vi "LHF.DB.Mongo.Collection.DropIndex.vi"(8 "error in (no error)":errorcluster, 9 "value":variant, 10 "Collection":string, 11 "LHF.DB.Mongo in":refnum<class "LHF.DB.Mongo.lvclass">) -> (0 "error out":errorcluster, 1 "Ok":bool, 3 "LHF.DB.Mongo out":refnum<class "LHF.DB.Mongo.lvclass">)   [LabVIEW 2013, in "LHF.DB.Mongo.lvclass"]
doc: "Creates an index in collection. Variable name, type & content will be used."
uses:
  LHF.DB.Mongo.lvclass
  C:/Users/Ricardo/Desktop/Projetos/LabVIEW-MongoDB/src/Driver/MongoDB.Driver.dll
  LabVIEW-MongoDB/src/Driver/MongoDB.Driver.dll
  <vilib>/Utility/VariantDataType/VariantType.lvlib
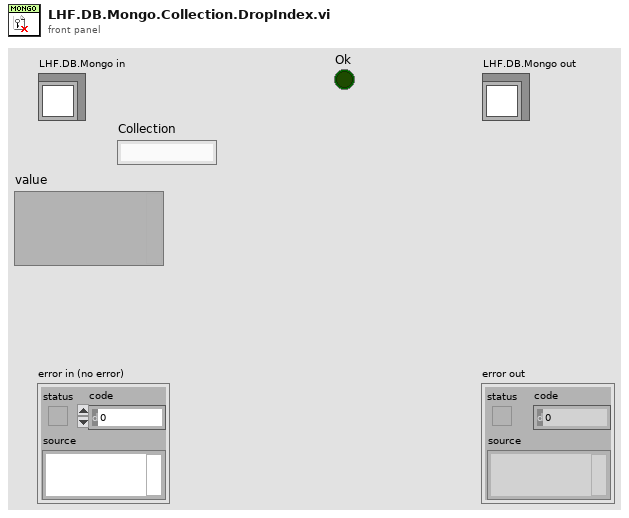
[diagram p1: front panel]
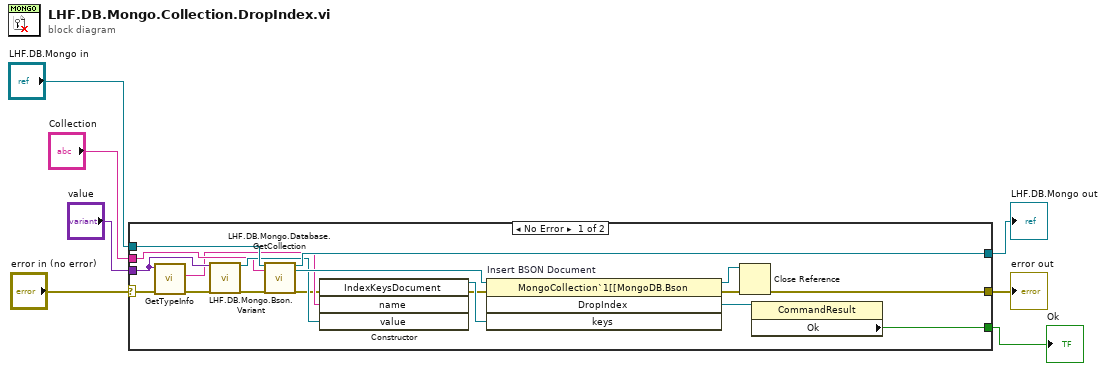
[diagram p0: block diagram]
diagram:
  n1 = case shown="No Error" "error in (no error)" {
    selector: "error in (no error)" -> [w13 w27]
    tunnel: [w10 w27] -> w6
    tunnel: [w23 w26] -> w4
    tunnel: "LHF.DB.Mongo in" -> [w24 w26]
    tunnel: "value" -> [w16 _]
    tunnel: "Collection" -> [w18 _]
    tunnel: [w8 _] -> w1
    frame No Error {
      n2 = call <vilib>:"GetTypeInfo.vi"("error in (no error)"=w13, "Variant"=w16) -> ("error out"=w14:errorcluster, "Name"=w15:string)  [unwired: 5 in, 3 out]
      n3 = call "LHF.DB.Mongo.Bson.Variant.vi"("Variant"=w16, "error IO"=w14) -> ("BsonValue"=w21:refnum<k24>, "error IO 2"=w12:errorcluster)  [unwired: 16 in]
      n4 = call "LHF.DB.Mongo.Database.GetCollection.vi"("LHF.DB.Mongo in"=w24, "collectionName"=w18, "error in (no error)"=w12) -> ("LHF.DB.Mongo in"=w23:refnum<class "LHF.DB.Mongo.lvclass">, "MongoCollection"=w22:refnum<k24>, "error out"=w11:errorcluster)  [unwired: 14 in]
      n5 = constructor class="IndexKeysDocument"(error in=w11, "name"=w15, "value"=w21) -> (reference out=w25:refnum<k24>, error out=w20:errorcluster)  [unwired: 2 in, 3 out]
      n6 = invoke on="Insert BSON Document" class="MongoCollection`1[[MongoDB.Bson" method="DropIndex"(reference=w22, error in=w20, "keys"=w25) -> (reference out=w17:refnum<k24>, error out=w19:errorcluster, "DropIndex"=w9:refnum<k24>)  [unwired: 1 in, 1 out]
      n7 = Close Reference(reference=w17, error in (no error)=w19) -> (error out=w10:errorcluster)
      n8 = property class="CommandResult"(reference=w9) -> ("Ok"=w8:bool)  [unwired: 1 in, 2 out]
    }
    frame Error {
    }
  }
  "error out" <- w6
  "LHF.DB.Mongo out" <- w4
  "Ok" <- w1
